vi "IMAQdx_setAttribute_U32.vi"(4 "error in (no error)":errorcluster, 5 "Value (U32)":u32, 6 "Attribute Name":string, 7 "IMAQdx Session":T1) -> (0 "error out":errorcluster, 1 "In Range?":bool, 3 "dup IMAQdx Session":T1)   [LabVIEW 2014, in "HGF_VisionTools.lvlib"]
doc: "This VI sets IMAQdx attribute value of type U32."
uses:
  HGF_VisionTools.lvlib
  <resource>/objmgr/imaqdx.rc
  HGF_LVC/HGF_Auxiliary/HGF_Auxiliary.lvlib
  HGF_LVC/HGF_Auxiliary/Severity.ctl
  HGF_LVC/HGF_Auxiliary/ErrorCode.ctl
  <vilib>/userdefined/High Color/IMAQdx.ctl
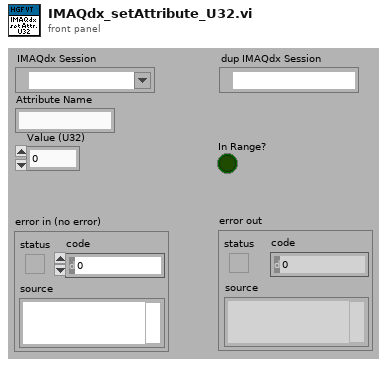
[diagram p1: front panel]
types:
  T1 = typedef "IMAQdx.ctl" = refnum<k21>
  T2 = typedef "HGF_Auxiliary.lvlib/ErrorCode.ctl" = enum32{"No error", "Function not supported.", "This VI is for friends only.", "Reference object aready exisits.", "Parameter out of range.", "Not a rendezvous.", "Invalid notifier reference.", "Invalid queue reference.", "Self-Test not supported.", "Reset not supported.", "IDN query not supported.", "Error query not supported.", "Incorrect addressee.", "Object already exists.", "No class name specified", "Driver not supported", "Attribute is not writable"}
  T3 = typedef "HGF_Auxiliary.lvlib/Severity.ctl" = enum16{"Info", "Warning", "Fault", "Error", "Fatal"}
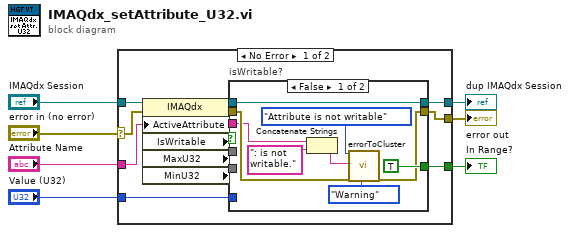
[diagram p0: block diagram]
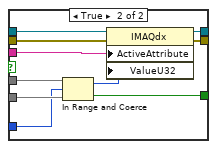
[diagram p2: hidden frame]
diagram:
  n1 = case shown="No Error" "error in (no error)" {
    selector: "error in (no error)" -> [w9 w39]
    tunnel: "IMAQdx Session" -> [w19 w40]
    tunnel: "Attribute Name" -> [w16 _]
    tunnel: "Value (U32)" -> [w13 _]
    tunnel: [w12 w40] -> w4
    tunnel: [w11 w39] -> w3
    tunnel: [w10 _] -> w2
    frame No Error {
      n2 = property class="IMAQdx"(reference=w19, error in=w9, "ActiveAttribute"=w16) -> (reference out=w18:T1, error out=w17:errorcluster, "IsWritable"=w8, "MaxU32"=w14, "MinU32"=w15)
      n3 = case "isWritable?" shown="False" w8 {
        tunnel: w18 -> [w28 w38]
        tunnel: w17 -> [w26 w37]
        tunnel: w16 -> [w22 w36]
        tunnel: w15 -> [_ w35]
        tunnel: w14 -> [_ w34]
        tunnel: w13 -> [_ w33]
        tunnel: [w28 w31] -> w12
        tunnel: [w25 w30] -> w11
        tunnel: [TRUE w29] -> w10
        frame False {
          n4 = Concatenate Strings(w22, ": is not writable." ("string")) -> (w20:string)
          n5 = call "errorToCluster.vi"("error code"=ErrorCode."Attribute is not writable", "error message (\"\")"=w20, "error in (no error)"=w26, "severity (Error)"=Severity."Warning") -> ("error out"=w25:errorcluster)  [unwired: 15 in]
        }
        frame True {
          n6 = In Range and Coerce(upper limit=w34, x=w33, lower limit=w35) -> (coerced(x)=w32:u32, In Range?=w29:bool)
          n7 = property class="IMAQdx"(reference=w38, error in=w37, "ActiveAttribute"=w36, "ValueU32"=w32) -> (reference out=w31:T1, error out=w30:errorcluster)
        }
      }
    }
    frame Error {
    }
  }
  "dup IMAQdx Session" <- w4
  "error out" <- w3
  "In Range?" <- w2
